vi "CANWrite.vi"(0 "Data1":u8, 1 "Data2":u8, 2 "Data3":u8, 5 "Data0":u8, 7 "ID_ToSend":u32, 9 "Data4":u8, 11 "Data5":u8, 12 "Data6":u8, 13 "Data7":u8) -> (8 "Frame":u32[](array[numeric]))   [LabVIEW 2013]
panel:
  # "以下均是十进制"
  # "如果ID的29位（共32位，从0开始）置1则表示扩展帧，或者表示标准帧"
  # "数据长度"
  # "8字节数据场"
  # "此处生成的6个32位数字构成的数组直接输入CAN总线即可传输"
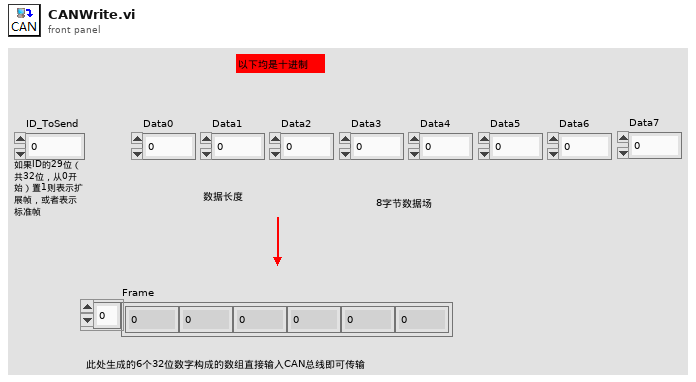
[diagram p1: front panel]
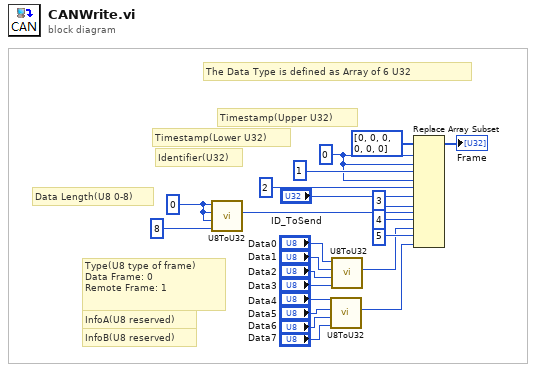
[diagram p0: block diagram]
diagram:
  w15 = u8 0 ("x")
  w2 = 0 ("index")
  # "Data Length(U8 0-8)"
  # "InfoB(U8 reserved)"
  # "InfoA(U8 reserved)"
  # "Type(U8 type of frame) \nData Frame: 0\nRemote Frame: 1"
  # "Identifier(U32)"
  # "Timestamp(Lower U32)"
  # "Timestamp(Upper U32)"
  # "The Data Type is defined as Array of 6 U32"
  n1 = call "U8ToU32.vi"("x 4"=u8 8, "x 3"=w15, "x 2"=w15, "x"=w15) -> ("result"=w13:u32)  [unwired: 7 in]
  n2 = call "U8ToU32.vi"("x 4"="Data7", "x 3"="Data6", "x 2"="Data5", "x"="Data4") -> ("result"=w3:u32)  [unwired: 7 in]
  n3 = call "U8ToU32.vi"("x 4"="Data3", "x 3"="Data2", "x 2"="Data1", "x"="Data0") -> ("result"=w8:u32)  [unwired: 7 in]
  n4 = Replace Array Subset(array=u32[] [0, 0, 0, 0, 0, 0] ("Array"), new element #1=w2, index #1=w2, new element #2=w2, index #2=1 ("index"), new element #3="ID_ToSend", index #3=2 ("index"), new element #4=w13, index #4=3 ("index"), new element #5=w8, index #5=4 ("index"), new element #6=w3, index #6=5 ("index")) -> (→"Frame":u32[])
